vi "Map symbols.vi"(10 "Input Bit Stream":i8[](array[numeric]), 11 "Symbol Map":cdb[](array[numeric]) format="%.3f") -> (3 "Symbols":cdb[](array[numeric]) format="%.2f")   [LabVIEW 2011]
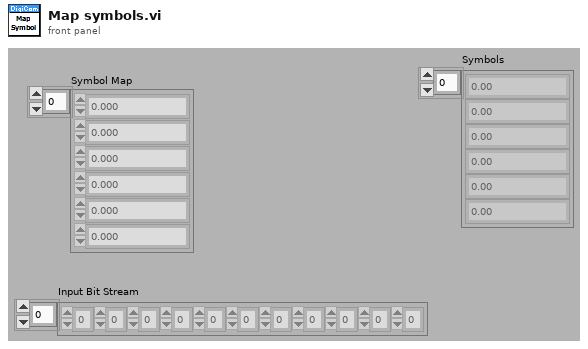
[diagram p1: front panel]
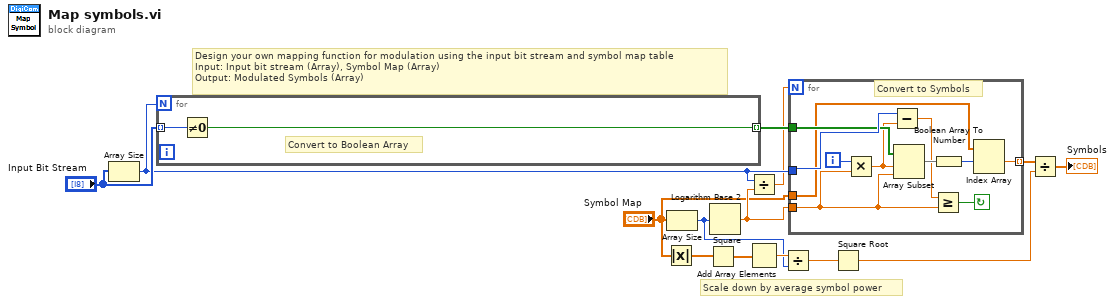
[diagram p0: block diagram]
diagram:
  # "Scale down by average symbol power"
  # "Design your own mapping function for modulation using the input bit stream and symbol map table\nInput: Input bit stream (Array), Symbol Map (Array)\nOutput: Modulated Symbols (Array)"
  n1 = Array Size(array="Input Bit Stream") -> (size(s)=w12:i32)
  n2 = for {
    N: w12 -> [_]
    tunnel: "Input Bit Stream" -> [w16] mode=indexing
    tunnel: [w15] -> w13 mode=indexing
    # "Convert to Boolean Array"
    n3 = Not Equal To 0?(x=w16) -> (x != 0?=w15:bool)
  }
  n4 = Absolute Value(x="Symbol Map") -> (abs(x)=w8:dbl[])
  n5 = Array Size(array="Symbol Map") -> (size(s)=w5:i32)
  n6 = Square(x=w8) -> (x^2=w7:dbl[])
  n7 = Logarithm Base 2(1:w5) -> (0:w11:dbl)
  n8 = Divide(x=w12, y=w11) -> (x/y=w10:dbl)
  n9 = Add Array Elements(numeric array=w7) -> (sum=w6:dbl)
  n10 = Divide(x=w6, y=w5) -> (x/y=w4:dbl)
  n11 = for {
    N: w10 -> [_]
    tunnel: w12 -> [w27]
    tunnel: w13 -> [w26]
    tunnel: w11 -> [w21]
    tunnel: "Symbol Map" -> [w22]
    tunnel: [w18] -> w3 mode=indexing
    i -> [w19]
    stop <- w17 continue-if-true
    # "Convert to Symbols"
    n12 = Multiply(x=w19, y=w21) -> (x*y=w25:dbl)
    n13 = Subtract(x=w27, y=w25) -> (x-y=w20:dbl)
    n14 = Array Subset(array=w26, index=w25, length=w21) -> (w24:bool[])
    n15 = Greater Or Equal?(x=w20, y=w21) -> (x >= y?=w17:bool)
    n16 = Boolean Array To Number(Boolean array=w24) -> (number=w23:u32)
    n17 = Index Array(array=w22, index #1=w23) -> (element #1=w18:cdb)  [unwired: 1 in, 1 out]
  }
  n18 = Square Root(x=w4) -> (sqrt(x)=w2:dbl)
  n19 = Divide(x=w3, y=w2) -> (x/y=→"Symbols":cdb[])
